vi "read metadata.vi"(8 "error in":errorcluster, 11 "system tag in":refnum<class "tag descriptor.lvclass">) -> (0 "error out":errorcluster, 2 "metadata":string, 3 "system tag out":refnum<class "tag descriptor.lvclass">)   [LabVIEW 2013, in "tag bus.lvlib" / "tag descriptor.lvclass"]
doc: "Reads the metadata field in a tag descriptor. This field can be used for any user-defined information, like a description."
uses:
  tag descriptor.lvclass
  tag descriptor.lvclass/tag descriptor.ctl
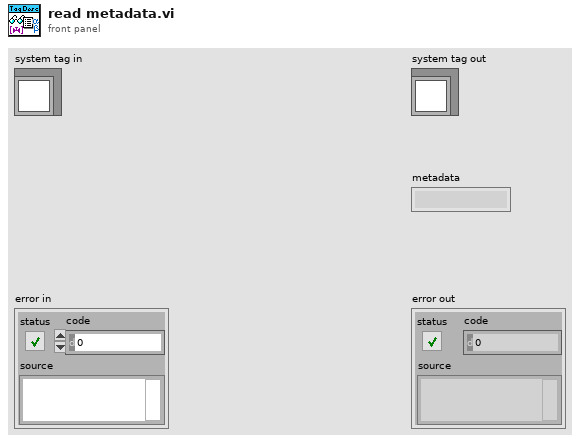
[diagram p1: front panel]
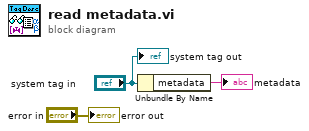
[diagram p0: block diagram]
diagram:
  n1 = Unbundle By Name("system tag in") -> ("metadata"=→"metadata":string)
  "system tag out" <- "system tag in"
  "error out" <- "error in"
